vi "Ordering_Type Write.vi"(4 "error in (no error)":errorcluster, 5 "Value":T2, 6 "Container State":T4, 7 "Display State In":T1) -> (0 "error out":errorcluster, 3 "Display State Out":T1)   [LabVIEW 2012, in "ListBox_XControl.xctl"]
uses:
  ListBox_XControl.xctl
  <vilib>/_xctls/Container State.ctl
  VIs/Order Type Def.ctl
  ListBox_State.ctl
  VIs/Value Filters.ctl
  <vilib>/_xctls/XControlSupport.lvlib
panel:
  # "Replace the Value Control below with a Control of desired type.\nDo not remove this Control or the others from the connector pane.\nDo not change the connector pane pattern.\nThe Value control should always be the third terminal from top on the input side in the connector pane."
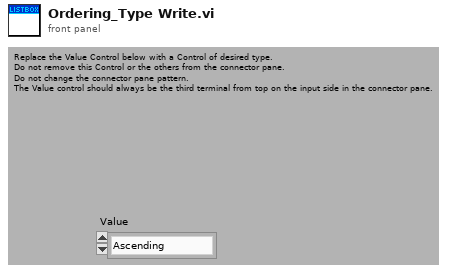
[diagram p1: front panel]
types:
  T1 = typedef "ListBox_XControl.xctl/ListBox_State.ctl" = cluster{"Alternating BG Color":u32, "Alternating Text Color":u32, "Order by Col":i32, "Order":T2, "Value Filters":T3, "Item Names before Filtering":string[][], "Item Names after Filtering":string[][], "Column Header Strings[]":string[], "Column Widths":u32[], "Autosize by Column":i32, "Autosize Activated?":bool, "Autosize Cell Padding":u32}
  T2 = typedef "ListBox_XControl.xctl/Order Type Def.ctl" = enum16{"Ascending", "Descending", "Off"}
  T3 = typedef "ListBox_XControl.xctl/Value Filters.ctl" = cluster{"Column":i32, "Only include Values From":string, "Only include Values to":string}[]
  T4 = typedef "XControlSupport.lvlib/Container State.ctl" = cluster{"Indicator?":bool, "Run Mode?":bool, " Refnum":refnum<vi>}
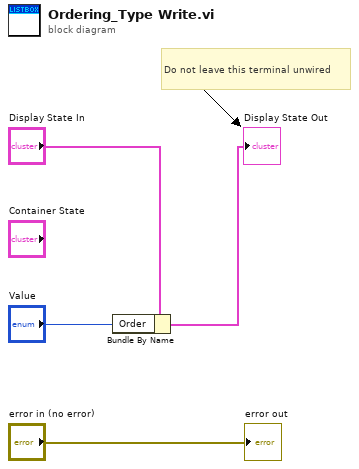
[diagram p0: block diagram]
diagram:
  # "Do not leave this terminal unwired"
  n1 = Bundle By Name(cluster="Display State In", "Order"="Value") -> (→"Display State Out":T1)
  "error out" <- "error in (no error)"
